vi "dbc-mark-signal.vi"(8 "error in (no error)":errorcluster, 9 "Numeric":i32=38, 10 "Array":string[](array[string]), 11 "dbc in":refnum<class "dbc.lvclass">) -> (0 "error out":errorcluster, 3 "dbc out":refnum<class "dbc.lvclass">)   [LabVIEW 2015, in "dbc.lvclass"]
uses:
  dbc.lvclass
  dbc.lvclass/dbc.ctl
  read-tree-ref.vi
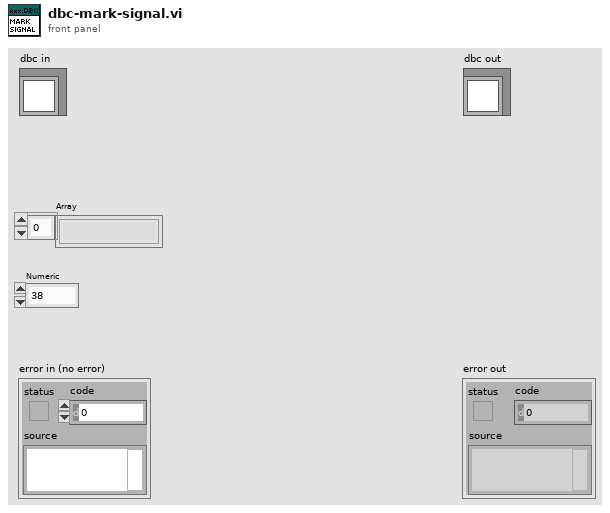
[diagram p1: front panel]
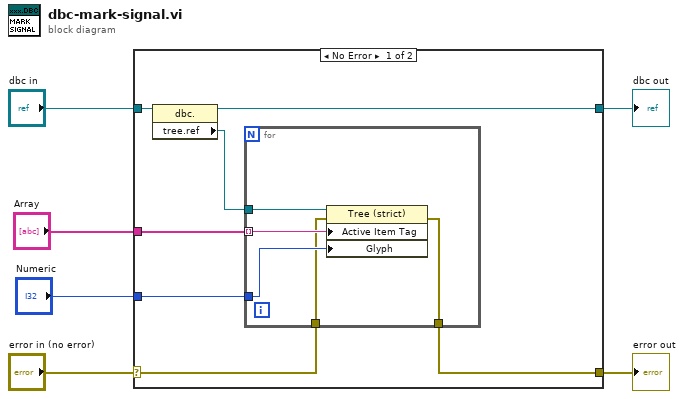
[diagram p0: block diagram]
diagram:
  n1 = case shown="No Error" "error in (no error)" {
    selector: "error in (no error)" -> [w8 w20]
    tunnel: [w7 w20] -> w5
    tunnel: [w12 w19] -> w3
    tunnel: "dbc in" -> [w13 w19]
    tunnel: "Array" -> [w10 _]
    tunnel: "Numeric" -> [w9 _]
    frame No Error {
      n2 = property class="dbc."(reference=w13) -> (reference out=w12:refnum<class "dbc.lvclass">, "tree.ref"=w11:refnum<vi>)  [unwired: 1 in, 1 out]
      n3 = for {
        tunnel: w11 -> [w18]
        tunnel: w10 -> [w17] mode=indexing
        tunnel: w9 -> [w16]
        tunnel: w8 -> [w15]
        tunnel: [w14] -> w7
        n4 = property class="Tree (strict)"(reference=w18, error in=w15, "Active Item Tag"=w17, "Glyph"=w16) -> (error out=w14:errorcluster)  [unwired: 1 out]
      }
    }
    frame Error {
    }
  }
  "error out" <- w5
  "dbc out" <- w3
